vi "Safety Elevator Mode.vi"(8 "Elevator Low":bool, 10 "Command":T1) -> (0 "Eject Out":bool, 1 "Finger Out":bool, 2 "output":dbl)   [LabVIEW 2014]
uses:
  Elevator Command.ctl
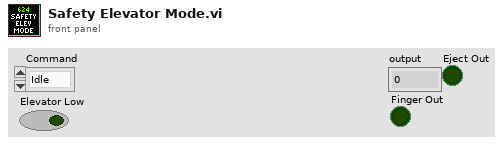
[diagram p1: front panel]
types:
  T1 = typedef "Elevator Command.ctl" = enum16{"Idle", "Load 1", "Load 2", "Load 3", "Drop Stack", "Eject Stack", "Load Trashcan"}
  T2 = enum16{"Idle", "Down", "Up", "Step Height", "Eject"}
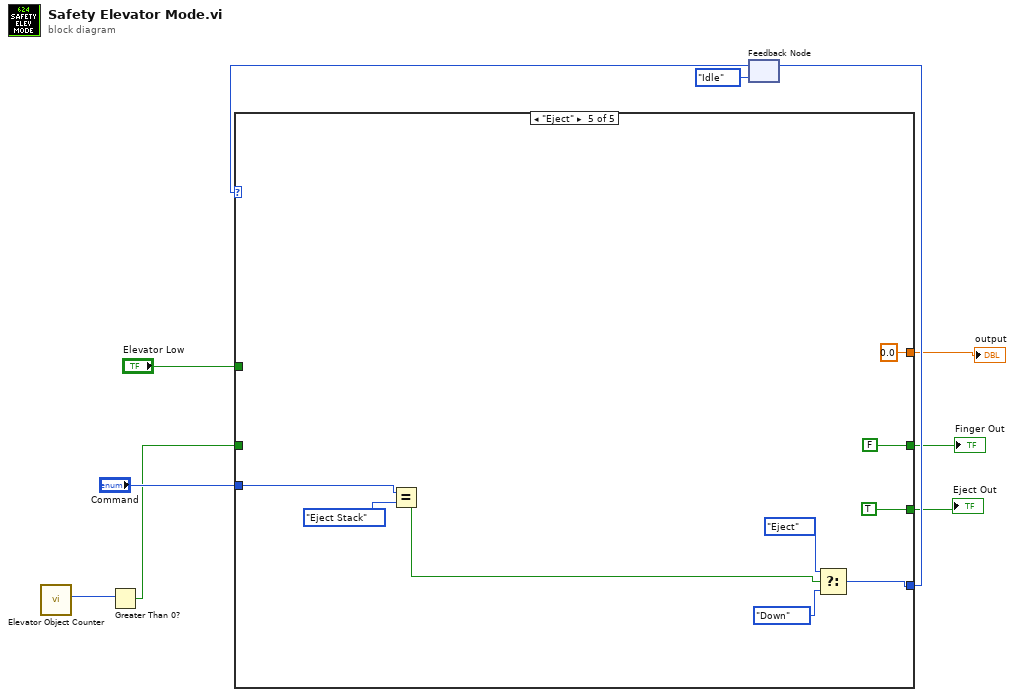
[diagram p0: block diagram]
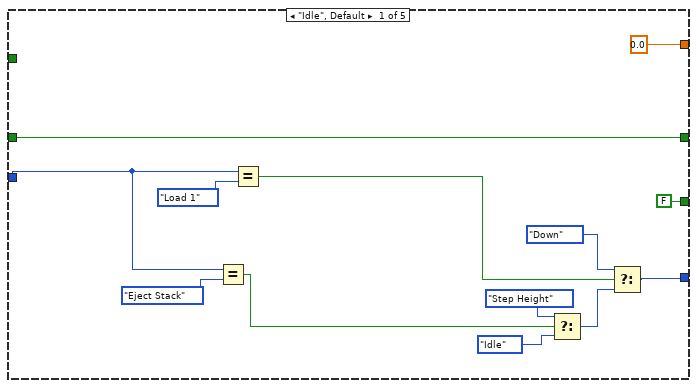
[diagram p2: hidden frame]
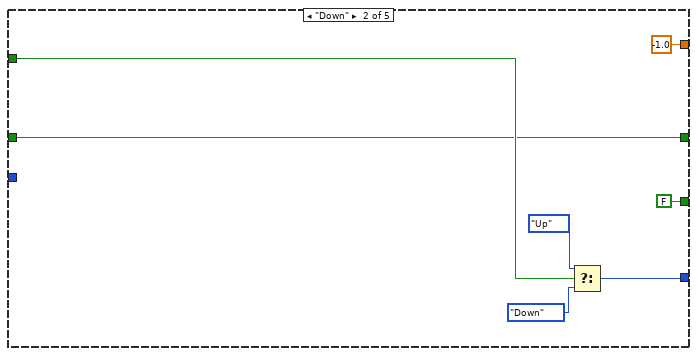
[diagram p3: hidden frame]
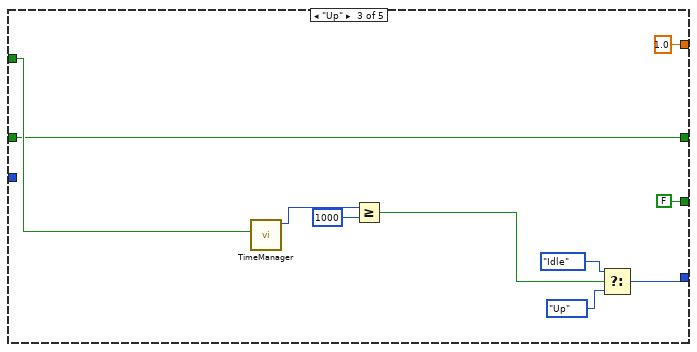
[diagram p4: hidden frame]
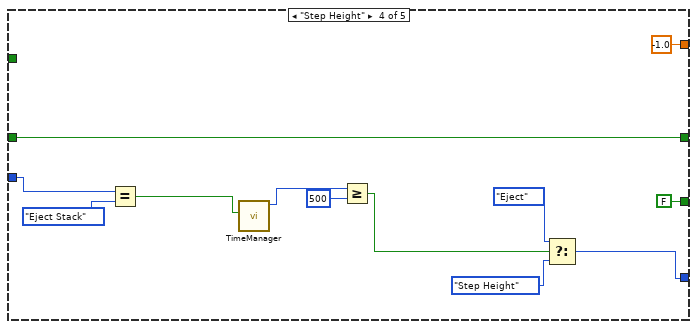
[diagram p5: hidden frame]
diagram:
  n1 = call "Elevator Object Counter.vi"() -> ("Tote Count"=w3:i8)  [unwired: 10 in, 1 out]
  n2 = Greater Than 0?(x=w3) -> (x > 0?=w2:bool)
  n3 = feedback #1(T2."Idle" ("Safety Elevator")) -> (w9:T2)
  n4 = case shown="\"Eject\"" w9 {
    tunnel: [w22 _ w39 w46 w59] -> w10
    tunnel: "Command" -> [w17 _ _ w45 w57]
    tunnel: "Elevator Low" -> [_ w29 w36 _ _]
    tunnel: [0.0 ("output") -1.0 ("output") 1.0 ("output") -1.0 ("output") 0.0 ("output")] -> w5
    tunnel: [_ w30 _ _ _] -> _
    tunnel: [FALSE ("Finger Out") FALSE ("Finger Out") FALSE ("Finger Out") FALSE ("Finger Out") TRUE ("Finger Out")] -> w4
    tunnel: [w11 w24 w31 w41 FALSE] -> w1
    tunnel: w2 -> [w11 w24 w31 w41 _]
    frame "Idle", Default {
      n5 = Equal?(x=w17, y=Elevator_Command."Eject Stack") -> (x = y?=w13:bool)
      n6 = Equal?(x=w17, y=Elevator_Command."Load 1") -> (x = y?=w21:bool)
      n7 = Select(t=T2."Step Height" ("Safety Elevator"), s=w13, f=T2."Idle" ("Safety Elevator")) -> (s? t:f=w14:T2)
      n8 = Select(t=T2."Down" ("Safety Elevator"), s=w21, f=w14) -> (s? t:f=w22:T2)
    }
    frame "Down" {
      n9 = Select(t=T2."Up" ("Safety Elevator"), s=w29, f=T2."Down" ("Safety Elevator")) -> (s? t:f=w30:T2)
    }
    frame "Up" {
      n10 = call "TimeManager.vi"("Reset?"=w36) -> ("Time Since Reset"=w35:u32)  [unwired: 9 in, 1 out]
      n11 = Greater Or Equal?(x=w35, y=u32 1000) -> (x >= y?=w33:bool)
      n12 = Select(t=T2."Idle" ("Safety Elevator"), s=w33, f=T2."Up" ("Safety Elevator")) -> (s? t:f=w39:T2)
    }
    frame "Step Height" {
      n13 = Equal?(x=w45, y=Elevator_Command."Eject Stack") -> (x = y?=w43:bool)
      n14 = call "TimeManager.vi"("Reset?"=w43) -> ("Time Since Reset"=w51:u32)  [unwired: 9 in, 1 out]
      n15 = Greater Or Equal?(x=w51, y=u32 500) -> (x >= y?=w47:bool)
      n16 = Select(t=T2."Eject" ("Safety Elevator"), s=w47, f=T2."Step Height" ("Safety Elevator")) -> (s? t:f=w46:T2)
    }
    frame "Eject" {
      n17 = Equal?(x=w57, y=Elevator_Command."Eject Stack") -> (x = y?=w56:bool)
      n18 = Select(t=T2."Eject" ("Safety Elevator"), s=w56, f=T2."Down" ("Safety Elevator")) -> (s? t:f=w59:T2)
    }
  }
  "output" <- w5
  "Finger Out" <- w1
  "Eject Out" <- w4
  n19 = feedback-in #1(w10) -> ()
